vi "PH_GUI_Class.constructor.vi"(0 "name":string, 2 "data in":string, 5 "error in":errorcluster) -> (14 "i ref out":refnum<vi>, 16 "data out":string, 19 "error out":errorcluster)   [LabVIEW 2014, in "PH_GUI_Class.lvlib"]
doc: "This class is forseen to be inherited from. With its help data of devices can be stored in the PHELIX shot data base (PSDB). \n\n\n\nauthor: Stefan Götte, GSI\n\nLicense Agreement for this software:\n\nCopyright (C)\nGesellschaft für Schwerionenforschung, GSI\nPlanckstr. 1\n64291 Darmstadt\nGermany\n\nContact: D.Beck@gsi.de \n\nThis program is free software; you can redistribute it and/or modify it under the terms of the \nGNU General Public License as published by the Free Software Foundation; either version 2 of \nthe license, or (at your option) any later version.\n\nThis program is distributed in the hope that it will be useful, but WITHOUT ANY WARRANTY; \nwithout even the implied warranty of MERCHANTABILITY or FITNESS FOR A PARTICULAR PURPOSE. See the GNU General License for more details (http://www.gnu.org).\n\nGesellschaft für Schwerionenforschung, GSI\nPlanckstr. 1, 64291 Darmstadt, Germany\nFor all questions and ideas contact: M.Richter@gsi.de, H.Brand@gsi.de or D.Beck@gsi.de.\nLast update: 16-JUN-2004"
uses:
  PH_GUI_Class.lvlib
  CS_Core/CSSystem/CSSystemLib/CSSystemLib.lvlib
  CS_Core/BaseGUI/BaseGUI.lvlib
  CS_Core/CSObj/CSObj.lvlib
  PH_Common/PH_Common.lvlib
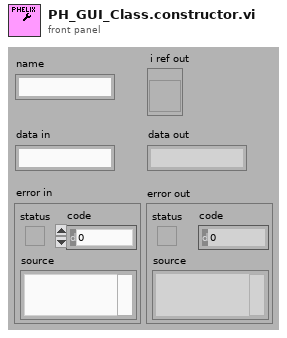
[diagram p1: front panel]
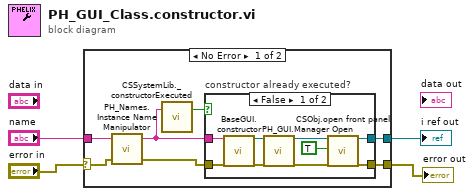
[diagram p0: block diagram]
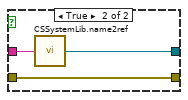
[diagram p2: hidden frame]
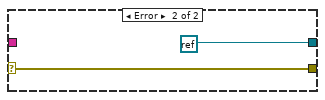
[diagram p3: hidden frame]
diagram:
  n1 = case shown="No Error" "error in" {
    selector: "error in" -> [w6 w24]
    tunnel: "name" -> [w8 _]
    tunnel: [w11 refnum<k0> refnum] -> w2
    tunnel: [w10 w24] -> w1
    frame No Error {
      n2 = call "PH_Names.Instance Name Manipulator.vi"("error in (no error)"=w6, "name in"=w8) -> ("error out"=w5:errorcluster, "name out"=w7:string)  [unwired: 1 in, 1 out]
      n3 = call "CSSystemLib._constructorExecuted.vi"("name"=w7) -> ("constructor executed?"=w9:bool)  [unwired: 18 in]
      n4 = case "constructor already executed?" shown="False" w9 {
        tunnel: [w16 w22] -> w11
        tunnel: [w17 w21] -> w10
        tunnel: w5 -> [w20 w21]
        tunnel: w7 -> [w19 w23]
        frame False {
          n5 = call "BaseGUI.constructor.vi"("name"=w19, "error in (no error)"=w20) -> ("i ref out"=w15:refnum<vi>, "error out"=w14:errorcluster)  [unwired: 15 in, 1 out]
          n6 = call "PH_GUI.Manager Open.vi"("i ref in"=w15, "error in"=w14) -> ("i ref out"=w13:refnum<vi>, "error out"=w12:errorcluster)  [unwired: 16 in]
          n7 = call "CSObj.open front panel.vi"("i ref in"=w13, "frontPanelOpen"=TRUE ("front panel open"), "error in (no error)"=w12) -> ("i ref out"=w16:refnum<vi>, "error out"=w17:errorcluster)  [unwired: 15 in]
        }
        frame True {
          n8 = call "CSSystemLib.name2ref.vi"("name"=w23) -> ("obj refnum"=w22:refnum<vi>)
        }
      }
    }
    frame Error {
    }
  }
  "i ref out" <- w2
  "error out" <- w1
